vi "DriveVisionPath.vi"() -> ()   [LabVIEW 2018]
uses:
  FRC-2018/new-FRC-2018/Shared/RobotNeededPathData.ctl
panel:
  in  "Angle":dbl
  in  "Right Distance":dbl
  in  "Left Distance":dbl
  in  "RobotNeededPathData":T1={"Path"=[], "MaxVel"=0.0, "MaxAccel"=0.0, "Backwards?"=FALSE, "PointSpacing"=0.0, "LookaheadDist"=0.0, "Speed/Curve"=1.8, "SlowDistanceAtEnd"=12.0, "SlowSpeed"=15.0, "MaxDeAccel"=0.0} {"SlowSpeed" format="%#_13g"; "SlowDistanceAtEnd" format="%#_13g"; "Speed/Curve" format="%#_13g"}
  in  "DeltaY":dbl
  in  "DeltaX":dbl
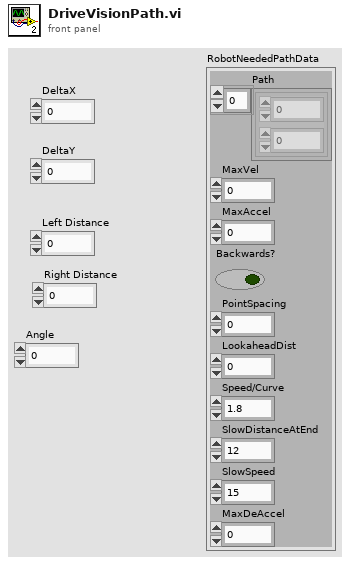
[diagram p1: front panel]
types:
  T1 = typedef "RobotNeededPathData.ctl" = cluster{"Path":cluster{dbl, dbl}[], "MaxVel":dbl, "MaxAccel":dbl, "Backwards?":bool, "PointSpacing":dbl, "LookaheadDist":dbl, "Speed/Curve":dbl, "SlowDistanceAtEnd":dbl, "SlowSpeed":dbl, "MaxDeAccel":dbl}
  T2 = cluster{"Path":cluster{dbl, dbl}[], "PointSpacing":dbl}
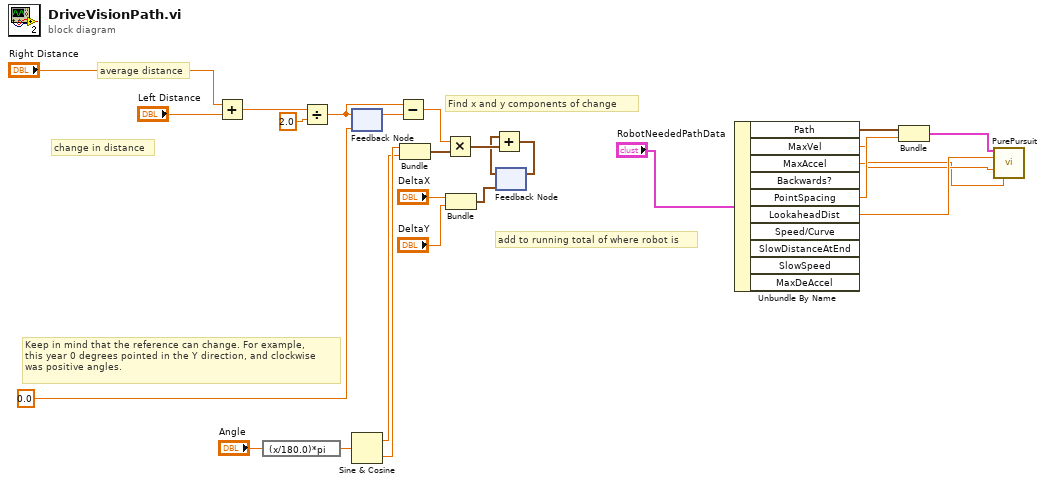
[diagram p0: block diagram]
diagram:
  # "Keep in mind that the reference can change. For example,\nthis year 0 degrees pointed in the Y direction, and clockwise\nwas positive angles."
  # "add to running total of where robot is"
  # "Find x and y components of change"
  # "change in distance"
  # "average distance"
  n1 = Add(x="Right Distance", y="Left Distance") -> (x+y=w18:dbl)
  n2 = expression code="(x/180.0)*pi" ("degrees to radians")("Angle") -> (w24:dbl)
  n3 = Divide(x=w18, y=2.0) -> (x/y=w17:dbl)
  n4 = feedback #1(0.0) -> (w26:dbl)
  n5 = feedback-in #1(w17) -> ()
  n6 = Sine & Cosine(0:w24) -> (1:w22:dbl, 2:w23:dbl)
  n7 = Subtract(x=w17, y=w26) -> (x-y=w20:dbl)
  n8 = Bundle(w23, w22) -> (w21:cluster{dbl, dbl})  [unwired: 1 in]
  n9 = Multiply(x=w20, y=w21) -> (x*y=w19:cluster{dbl, dbl})
  n10 = Bundle("DeltaX"="DeltaX", "DeltaY"="DeltaY") -> (w8:cluster{"DeltaX":dbl, "DeltaY":dbl})  [unwired: 1 in]
  n11 = feedback #2(w8) -> (w11:cluster{"DeltaX":dbl, "DeltaY":dbl})
  n12 = Add(x=w11, y=w19) -> (x+y=w12:cluster{dbl, dbl})
  n13 = feedback-in #2(w12) -> ()
  n14 = Unbundle By Name("RobotNeededPathData") -> ("Path"=w6:cluster{dbl, dbl}[], "MaxVel"=w2:dbl, "MaxAccel"=w1:dbl, "PointSpacing"=w5:dbl, "LookaheadDist"=w3:dbl)  [unwired: 5 out]
  n15 = Bundle("Path"=w6, "PointSpacing"=w5) -> (w4:T2)  [unwired: 1 in]
  n16 = call "PurePursuit.vi"("PathData"=w4, "LookAhead"=w3, "MaxVel"=w2, "Max Accel"=w1) -> ()  [unwired: 7 in, 5 out]
